vi "CreateBoard.vi"(8 "error in (no error)":errorcluster, 10 "Size":cluster{"Size":cluster{"X":i32, "Y":i32}}, 11 "Board in":refnum<class "Board_Game.lvclass">) -> (0 "error out":errorcluster, 3 "Board out":refnum<class "Board_Game.lvclass">)   [LabVIEW 2021, in "Board_Game.lvclass"]
uses:
  Board_Game.lvclass
  Board_Game.lvclass/Board_Game.ctl
panel:
  in  "Color Box":u32(colorbox)
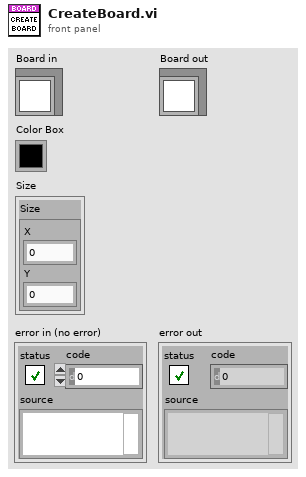
[diagram p1: front panel]
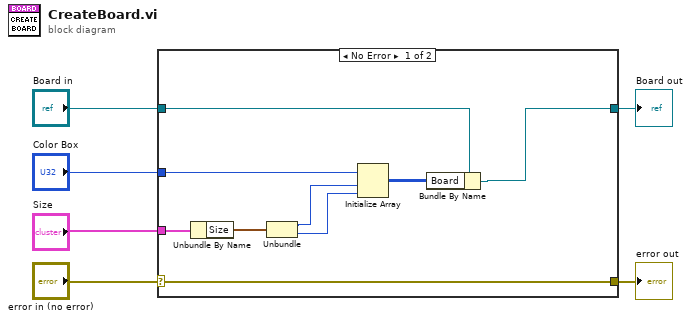
[diagram p0: block diagram]
diagram:
  n1 = case shown="No Error" "error in (no error)" {
    selector: "error in (no error)" -> [w15 w17]
    tunnel: [w15 w17] -> w5
    tunnel: [w9 w16] -> w3
    tunnel: "Board in" -> [w8 w16]
    tunnel: "Color Box" -> [w14 _]
    tunnel: "Size" -> [w13 _]
    frame No Error {
      n2 = Unbundle By Name(w13) -> ("Size"=w12:cluster{"X":i32, "Y":i32})
      n3 = Unbundle(w12) -> ("X"=w11:i32, "Y"=w7:i32)
      n4 = Initialize Array(w14, w11, w7) -> (w10:u32[][])
      n5 = Bundle By Name(cluster=w8, "Board"=w10) -> (w9:refnum<class "Board_Game.lvclass">)
    }
    frame Error {
    }
  }
  "error out" <- w5
  "Board out" <- w3
